vi "Simple UDP - Receiver.vi"() -> ()   [LabVIEW 2016]
doc: "The UDP protocol differs from TCP in that there is no error-checking with the packets of information that are sent, and thus no guarantee whatsoever that an intended recipient will actually receive a given piece of data.\n\nUDP does offer the ability to \"broadcast\" data across a network--simply specify an IP Address of all ones (255.255.255.255) to attempt to broadcast information network-wide. Keep in mind that routers and other network hardware will generally refuse to forward the broadcast beyond certain points, so the extent of the broadcast will in practice be limited."
panel:
  out "Received Data":dbl[][](graph)
  in  "Stop":bool
  # "Overview: Demonstrates the use of the UDP functions to receive data over a UDP connection.\nInstructions:\n1. Ensure Simple UDP - Sender.vi is already running.\n2. Run the VI.\n3. Click Stop to stop the VI."
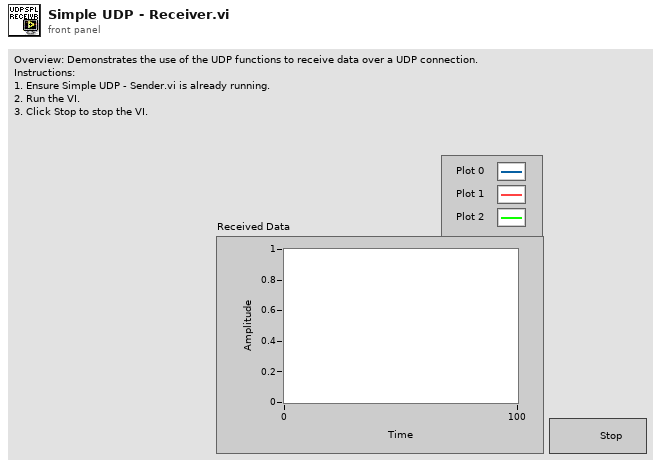
[diagram p1: front panel]
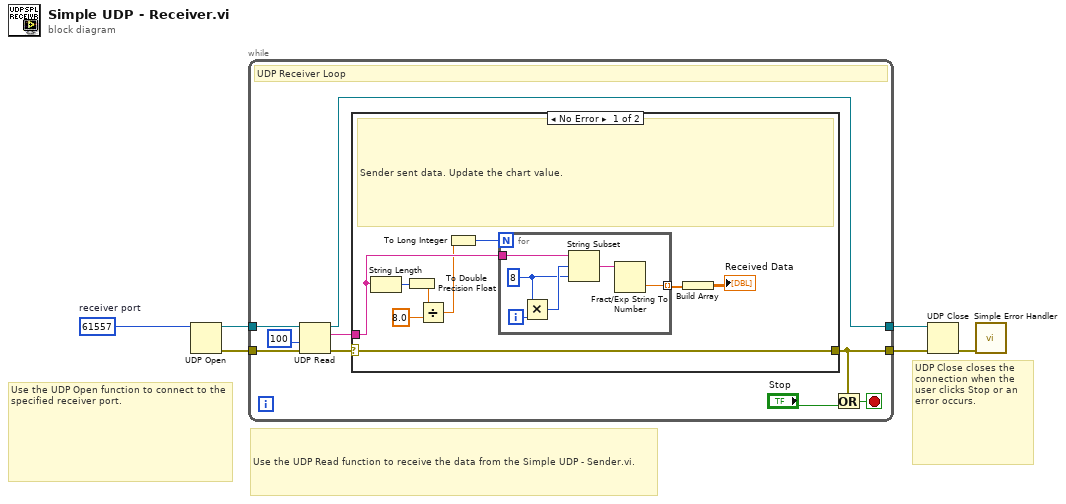
[diagram p0: block diagram]
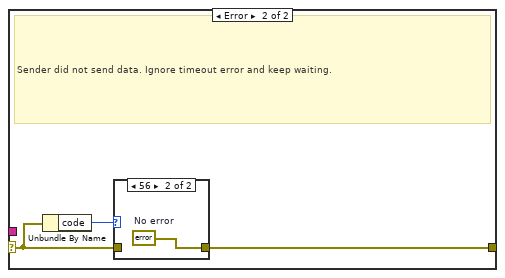
[diagram p2: hidden frame]
diagram:
  w1 = u16 61557  # receiver port
  # "UDP Close closes the connection when the user clicks Stop or an error occurs."
  # "Use the UDP Open function to connect to the specified receiver port."
  # "Use the UDP Read function to receive the data from the Simple UDP - Sender.vi."
  n1 = UDP Open(11:w1) -> (port=w2:refnum<k16>, 0:w3:errorcluster)  [unwired: 4 in, 1 out]
  n2 = while {
    tunnel: w2 -> [w15]
    tunnel: [w7] -> w6
    tunnel: w3 -> [w12]
    tunnel: [w8] -> w4
    stop <- w13 stop-if-true
    # "UDP Receiver Loop"
    n3 = UDP Read(connection ID=w15, timeout ms (25000)=100, 8:w12) -> (data out=w10:string, error out=w9:errorcluster, 3:w7:refnum<k16>)  [unwired: 3 out]
    n4 = case shown="No Error" w9 {
      selector: w9 -> [w24 w32]
      tunnel: w10 -> [w23 _]
      tunnel: [w24 w31] -> w8
      frame No Error {
        # "Sender sent data. Update the chart value."
        n5 = String Length(string=w23) -> (length=w19:i32)
        n6 = To Double Precision Float(number=w19) -> (double precision float=w18:dbl)
        n7 = Divide(x=w18, y=8.0 ("offset (0)")) -> (x/y=w20:dbl)
        n8 = To Long Integer(number=w20) -> (32bit integer=w21:i32)
        n9 = for {
          N: w21 -> [_]
          tunnel: w23 -> [w28]
          tunnel: [w30] -> w17 mode=indexing
          i -> [w29]
          w25 = 8 ("offset (0)")
          n10 = Multiply(x=w25, y=w29) -> (x*y=w26:i32)
          n11 = String Subset(string=w28, offset (0)=w26, length (rest)=w25) -> (substring=w27:string)
          n12 = Fract/Exp String To Number(string=w27) -> (number=w30:dbl)  [unwired: 3 in, 1 out]
        }
        n13 = Build Array(w17) -> (→"Received Data":dbl[][])
      }
      frame Error {
        # "Sender did not send data. Ignore timeout error and keep waiting."
        n14 = Unbundle By Name(w32) -> ("code"=w33:i32)
        n15 = case shown="56" w33 {
          tunnel: w32 -> [w34 _]
          tunnel: [w34 w35] -> w31
          frame Default {
          }
          frame 56 {
            w35 = errorcluster {"status"=FALSE, "code"=0, "source"=""}  # No error
          }
        }
      }
    }
    n16 = Or(x=w8, y="Stop") -> (x .or. y?=w13:bool)
  }
  n17 = UDP Close(connection ID=w6, 8:w4) -> (error out=w5:errorcluster)  [unwired: 1 out]
  n18 = call <vilib>:"Simple Error Handler.vi"("error in (no error)"=w5) -> ()  [unwired: 1 in, 8 out]
